vi "test Required Buffer Size.vi"(8 "error in (no error)":errorcluster, 11 "TestCase in":refnum<class "Configuration Tests.lvclass">) -> (0 "error out":errorcluster, 3 "TestCase out":refnum<class "Configuration Tests.lvclass">)   [LabVIEW 2017, in "Configuration Tests.lvclass"]
uses:
  Configuration Tests.lvclass
  Mock Classes/Transfer/Mock Transfer.lvclass
  C:/github/data-sharing-framework/Data Sharing Framework Core/Engine/Classes/Transfer/Transfer.lvclass
  Configuration/Public/Controls/DSF Engine Channel Configuration.ctl
  Configuration/Public/Controls/DSF Data Type.ctl
  Mock Classes/Transfer Group/Mock Transfer Group.lvclass
  C:/github/data-sharing-framework/Data Sharing Framework Core/Engine/Classes/Transfer Group/Transfer Group.lvclass
  <vilib>/addons/_JKI Toolkits/VI Tester/TestCase.llb/TestCase.lvclass
  Engine/Classes/Transfer Group/Transfer Group.lvclass
  Engine/Classes/Transfer/Transfer.lvclass
  DSF Core.lvlib
  C:/Program Files (x86)/National Instruments/LabVIEW 2017/vi.lib/addons/_JKI Toolkits/VI Tester/TestCase.llb/TestCase.lvclass
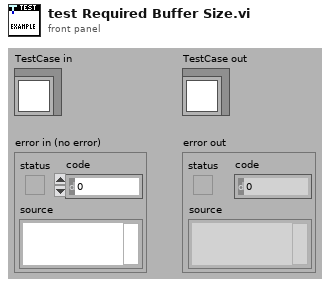
[diagram p1: front panel]
types:
  T1 = typedef "DSF Core.lvlib/DSF Engine Channel Configuration.ctl" = cluster{"engine offset":u64, "name":string, "data type":T2, "count":u64, "buffer offset":u64}
  T2 = typedef "DSF Core.lvlib/DSF Data Type.ctl" = enum8{"Bool", "SGL", "DBL", "I8", "I16", "I32", "I64", "U8", "U16", "U32", "U64"}
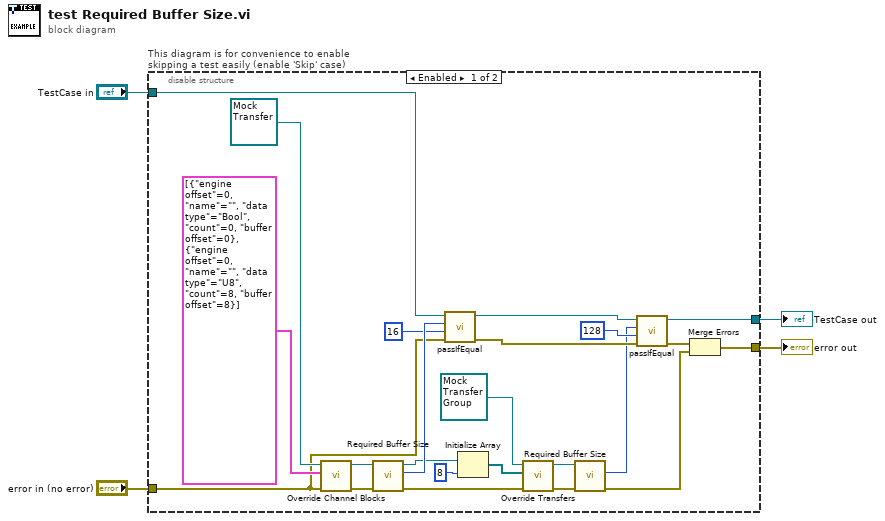
[diagram p0: block diagram]
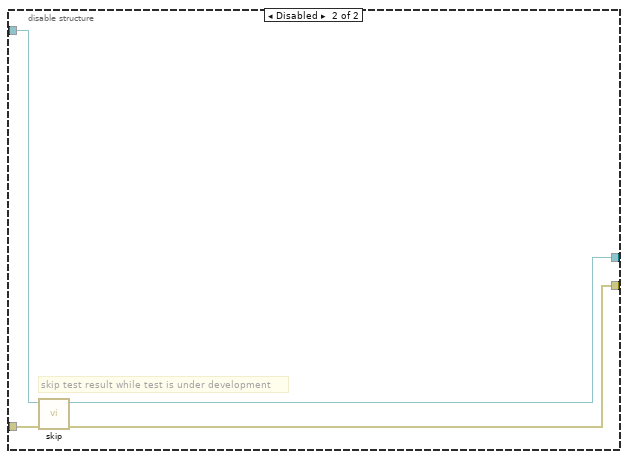
[diagram p2: hidden frame]
diagram:
  n1 = disable-structure "This diagram is for convenience to enable skipping a test easily (enable 'Skip' case)" shown="Enabled" {
    disable-tunnel: "TestCase in" -> [w23 w31]
    disable-tunnel: [w13 w29] -> w1
    disable-tunnel: [w7 w30] -> w3
    disable-tunnel: "error in (no error)" -> [w5 w28]
    frame Enabled {
      n2 = call "Override Channel Blocks.vi"("error in (no error)"=w5, "channel blocks"=T1[] [{"engine offset"=0, "name"="", "data type"=enum."Bool", "count"=0, "buffer offset"=0}, {"engine offset"=0, "name"="", "data type"=enum."U8", "count"=8, "buffer offset"=8}], "Mock Transfer in"=refnum<class "Mock Transfer.lvclass"> refnum ("Mock Transfer.lvclass")) -> ("error out"=w10:errorcluster, "Mock Transfer out"=w25:refnum<class "Mock Transfer.lvclass">)  [unwired: 7 in]
      n3 = call "Required Buffer Size.vi"("error in (no error)"=w10, "Transfer in"=w25) -> ("error out"=w9:errorcluster, "required buffer size"=w22:u64, "Transfer out"=w20:refnum<class "Mock Transfer.lvclass">)  [unwired: 7 in]
      n4 = call-dynamic "passIfEqual.vi"("error in (no error)"=w5, "y"=u64 16 ("required buffer size"), "x"=w22, "TestCase in"=w23) -> ("error out"=w24:errorcluster, "TestCase out"=w14:refnum<class "Configuration Tests.lvclass">)  [unwired: 6 in]
      n5 = Initialize Array(w20, 8 ("dimension size")) -> (w18:refnum<class "Mock Transfer.lvclass">[])
      n6 = call "Override Transfers.vi"("error in (no error)"=w9, "Transfers"=w18, "Mock Transfer Group in"=refnum<class "Mock Transfer Group.lvclass"> refnum) -> ("error out"=w8:errorcluster, "Mock Transfer Group out"=w17:refnum<class "Mock Transfer Group.lvclass">)  [unwired: 7 in]
      n7 = call "Required Buffer Size.vi"("error in (no error)"=w8, "Transfer Group in"=w17) -> ("error out"=w6:errorcluster, "required buffer size"=w11:u64)  [unwired: 7 in, 1 out]
      n8 = call-dynamic "passIfEqual.vi"("error in (no error)"=w24, "y"=u64 128 ("required buffer size"), "x"=w11, "TestCase in"=w14) -> ("error out"=w15:errorcluster, "TestCase out"=w13:refnum<class "Configuration Tests.lvclass">)  [unwired: 6 in]
      n9 = Merge Errors(w15, w6) -> (w7:errorcluster)
    }
    frame Disabled {
      # "skip test result while test is under development"
      n10 = call <vilib>:"skip.vi"("error in (no error)"=w28, "TestCase in"=w31) -> ("error out"=w30:errorcluster, "TestCase out"=w29:refnum<class "Configuration Tests.lvclass">)  [unwired: 8 in]
    }
  }
  "error out" <- w3
  "TestCase out" <- w1
